vi "Финал (6).vi"() -> ()   [LabVIEW 2017]
panel:
  in  "C":bool
  in  "Reset Out":bool
  in  "Reset Memory":bool
  in  "Reset":bool
  in  "adr B":cluster{"B 0":bool, "B 1":bool}
  in  "adr A":cluster{"A 0":bool, "A 1":bool}
  in  "Dec":T1
  out "Digs":T2
  out "L":T3
  out "Flags":T4
  in  "K":T5
  # "15-11+9-5"
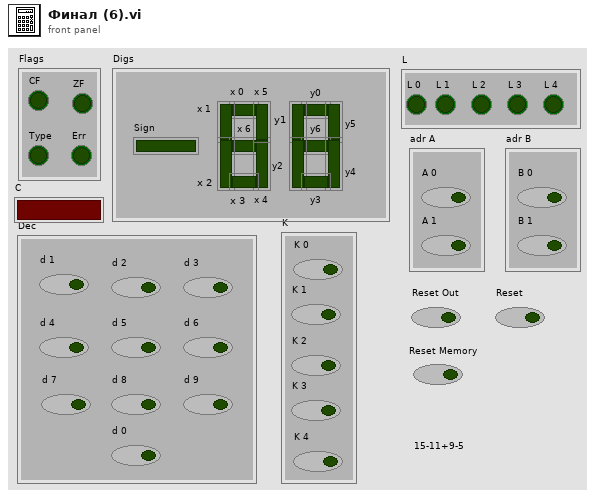
[diagram p1: front panel]
types:
  T1 = cluster{"d 0":bool, "d 1":bool, "d 2":bool, "d 3":bool, "d 4":bool, "d 5":bool, "d 6":bool, "d 7":bool, "d 8":bool, "d 9":bool}
  T2 = cluster{"y0":bool, "y1":bool, "y5":bool, "y6":bool, "y2":bool, "y4":bool, "y3":bool, "x 0":bool, "x 1":bool, "x 6":bool, "x 4":bool, "x 2":bool, "x 5":bool, "x 3":bool, "Sign":bool}
  T3 = cluster{"L 0":bool, "L 1":bool, "L 2":bool, "L 3":bool, "L 4":bool}
  T4 = cluster{"CF":bool, "ZF":bool, "Type":bool, "Err":bool}
  T5 = cluster{"K 0":bool, "K 1":bool, "K 2":bool, "K 3":bool, "K 4":bool}
  T6 = cluster{"c 0":bool, "c 1":bool, "c 2":bool, "c 3":bool, "c 4":bool}
  T7 = cluster{"L0":bool, "L1":bool, "L2":bool, "L3":bool, "L4":bool}
  T8 = cluster{"Y0":bool, "Y1":bool, "Y5":bool, "Y6":bool, "Y\n2":bool, "Y4":bool, "Y3":bool, "X0":bool, "X1":bool, "X6":bool, "X4":bool, "X2":bool, "X5":bool, "X3":bool, "Sign":bool}
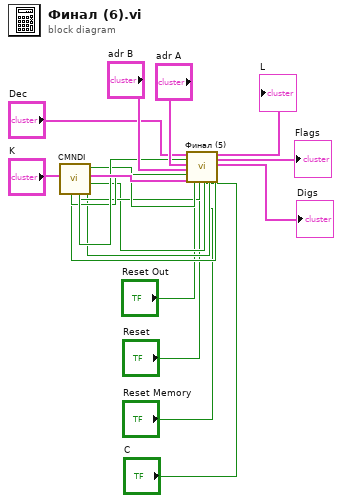
[diagram p0: block diagram]
diagram:
  n1 = call "CMNDI.vi"("K"="K") -> ("ClearAcc"=w9:bool, "Exec"=w10:bool, "Func"=w18:T6, "SelOp"=w12:bool, "Cread"=w14:bool, "Wr"=w11:bool, "Read"=w8:bool, "SelInp"=w13:bool)  [unwired: 3 in]
  n2 = call "Финал (5).vi"("Dec"="Dec", "Cread"=w14, "adr A"="adr A", "adr B"="adr B", "SelInp"=w13, "C Func"=w18, "SelOp"=w12, "Reset Out"="Reset Out", "WR"=w11, "Reset"="Reset", "C"="C", "Exec"=w10, "Reset Memory"="Reset Memory", "ClearAcc"=w9, "Read"=w8) -> ("L"=→"L":T7, "Flags"=→"Flags":T4, "Digs"=→"Digs":T8)  [unwired: 2 in]
